vi "配置文件项-未实现.vi"(8 "error out":errorcluster={"status"=TRUE, "code"=0, "source"=""}) -> (0 "输出簇":errorcluster)   [LabVIEW 2017]
panel:
  in  "键名":string
  in  "段名":string
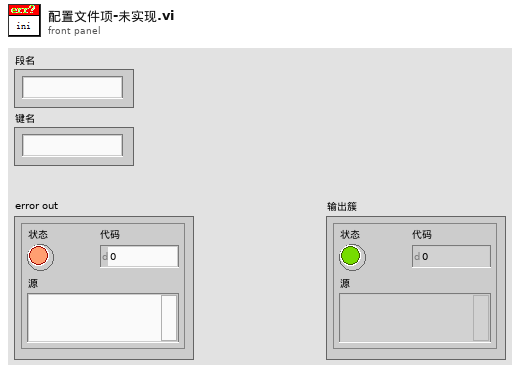
[diagram p1: front panel]
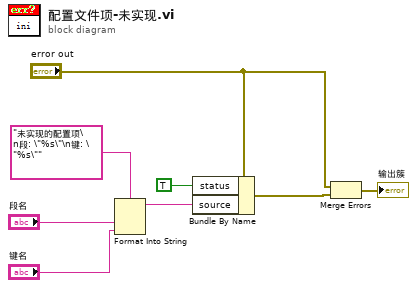
[diagram p0: block diagram]
diagram:
  n1 = Format Into String(format string="未实现的配置项\n段: \"%s\"\n键: \"%s\"" ("格式字符串"), "段名", "键名") -> (resulting string=w6:string)  [unwired: 2 in, 1 out]
  n2 = Bundle By Name(cluster="error out", "status"=TRUE, "source"=w6) -> (w3:errorcluster)
  n3 = Merge Errors("error out", w3) -> (→"输出簇":errorcluster)
